vi "SVPO Single Block Integration (1 Ch DBL WDT).vi"(7 "desired base units for length":i32(ring) items=["no change"=-1, "m"=0, "mm"=2, "microns"=3, "in"=1, "mils"=5], 9 "known condition":T1={"condition type"=enum."Initial Value", "known value"=nan}, 11 "scaled signal [EU]":waveform(dbl)) -> (3 "integrated signal [EU*s]":waveform(dbl))   [LabVIEW 2017, in "SoundVib_Integration.lvlib"]
doc: "Converts acceleration to velocity or velocity to displacement using a time-domain waveform as the input. Wire data to the <B>scaled signal [EU]</B> input to determine the polymorphic instance to use or manually select the instance. This VI performs Single Integration only. You can pass the integrated signal [EU*s] output to the scaled signal [EU] input of second call to this VI to perform double integration."
uses:
  <vilib>/addons/Sound and Vibration/svt_Integration/SoundVib_Integration.lvlib
  <vilib>/addons/_NISVFA/_Shared subVIs/Controls/svc_Integration Known Condition.ctl
  <vilib>/Analysis/2dsp.llb/Integral x(t).vi
  <vilib>/Analysis/baseanly.llb/Mean.vi
  <vilib>/Analysis/baseanly.llb/Mean (DBL).vi
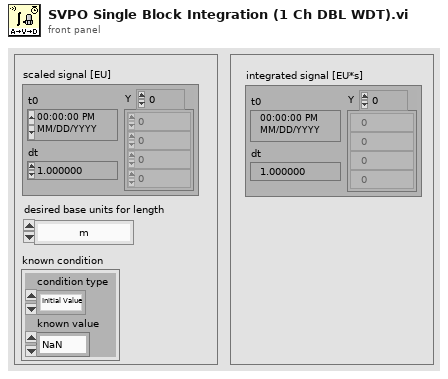
[diagram p1: front panel]
types:
  T1 = typedef "svc_Integration Known Condition.ctl" = cluster{"condition type":enum16{"Initial Value", "Mean Value", "Final Value"}, "known value":dbl}
  T2 = enum16{"single integration", "double integration"}
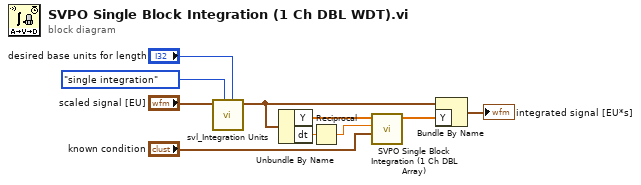
[diagram p0: block diagram]
diagram:
  n1 = call <vilib>:"svl_Integration Units.vi"("desired base units for length"="desired base units for length", "integration type"=T2."single integration", "scaled signal [EU]"="scaled signal [EU]") -> ("scaled signal out"=w2:waveform(dbl))  [unwired: 6 in, 2 out]
  n2 = Unbundle By Name(w2) -> ("Y"=w8:dbl[], "dt"=w10:dbl)
  n3 = Reciprocal(x=w10) -> (1/x=w9:dbl)
  n4 = call <vilib>:"SVPO Single Block Integration (1 Ch DBL Array).vi"("known condition"="known condition", "sampling rate [Hz]"=w9, "scaled signal [EU]"=w8) -> ("integrated signal [EU*s]"=w6:dbl[])  [unwired: 8 in]
  n5 = Bundle By Name(cluster=w2, "Y"=w6) -> (→"integrated signal [EU*s]":waveform(dbl))
